vi "Error Handler.vi"(4 "Error I64 [0]":i64, 5 "Label":string, 6 "Error I32 [0]":i32, 7 "Error if 0? [T]":bool=TRUE, 8 "error in (no error)":errorcluster) -> (0 "error out":errorcluster)   [LabVIEW 2018, in "LogonUser.lvclass"]
doc: "©2019\nWiebe Walstra\nwww.carya.nl"
uses:
  LogonUser.lvclass
  <vilib>/Utility/error.llb/Error Cluster From Error Code.vi
  <vilib>/ErrorRing/Error Ring.xnode
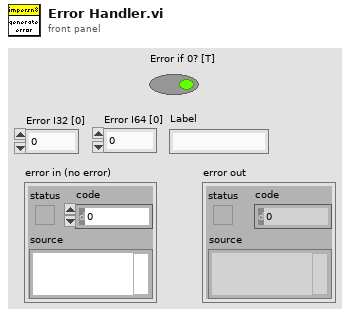
[diagram p1: front panel]
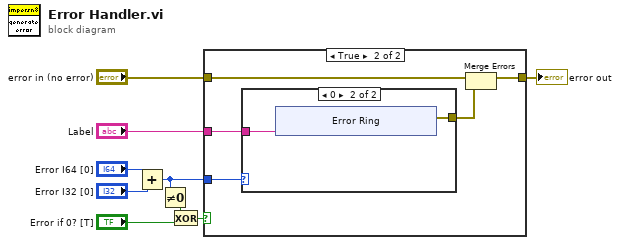
[diagram p0: block diagram]
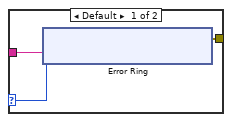
[diagram p3: hidden frame]
diagram:
  n1 = Add(x="Error I64 [0]", y="Error I32 [0]") -> (x+y=w1:i64)
  n2 = Not Equal To 0?(x=w1) -> (x != 0?=w7:bool)
  n3 = Exclusive Or(1:"Error if 0? [T]", 2:w7) -> (0:w6:bool)
  n4 = case shown="True" w6 {
    tunnel: "Label" -> [_ w15]
    tunnel: w1 -> [_ w14]
    tunnel: "error in (no error)" -> [w10 w13]
    tunnel: [w10 w11] -> w4
    frame False {
    }
    frame True {
      n5 = case shown="0" w14 {
        selector: w14 -> [w17 _]
        tunnel: w15 -> [w18 w28]
        tunnel: [w16 w27] -> w12
        frame Default {
          n6 = xnode "Error Ring"("parameter 0"=w18, "parameter 1"=w17) -> ("error out"=w16:errorcluster)
        }
        frame 0 {
          n7 = xnode "Error Ring"("parameter 0"=w28) -> ("error out"=w27:errorcluster)
        }
      }
      n8 = Merge Errors(w13, w12) -> (w11:errorcluster)
    }
  }
  "error out" <- w4
